vi "Test Gradient Control.vi"() -> ()   [LabVIEW 2015]
panel:
  in  "Frame Color":u32(colorbox)=16777216
  in  "Direction":T1(ring)
  in  "Slide":dbl(slide) scale=0.0..1.0
  in  "stop":bool
  in  "Color 2":u32(colorbox)
  in  "Color 1":u32(colorbox)
  out "Color Ramp":i32[][](graph)
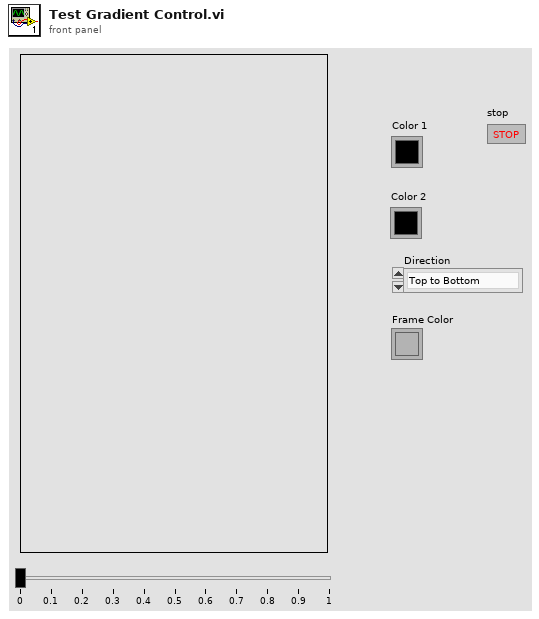
[diagram p1: front panel]
types:
  T1 = enum16{"Top to Bottom", "Bottom to Top", "Left to Right", "Right to Left"}
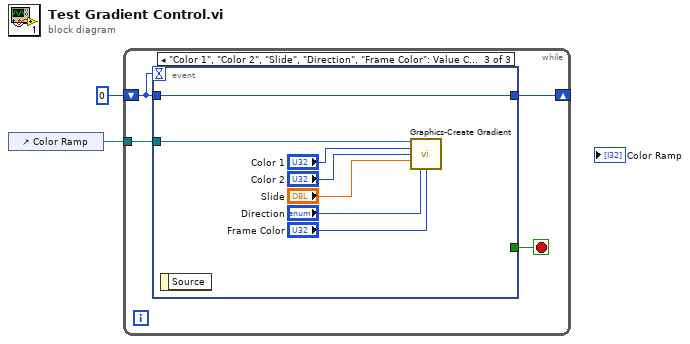
[diagram p0: block diagram]
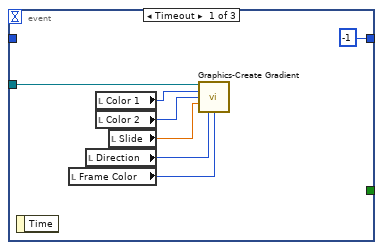
[diagram p2: hidden frame]
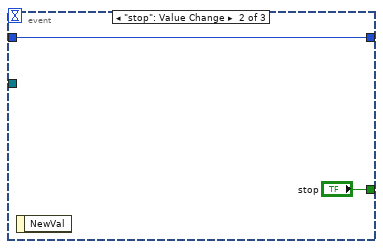
[diagram p3: hidden frame]
diagram:
  n1 = control-ref of="Color Ramp"() -> (w1:refnum<vi>)
  n2 = while {
    shift-right: [w4] -> _
    shift-left: 0 -> [w5]
    tunnel: w1 -> [w3]
    stop <- w6 stop-if-true
    n3 = event shown="[2] \"Color 1\", \"Color 2\", \"Slide\", \"Direction\", \"Frame Color\": Value Change" {
      selector: _ -> [_ _ _]
      dyn-events: _ -> [_ _ _]
      timeout: w5 -> [_ _ _]
      tunnel: [_ "stop" _] -> w6
      tunnel: w5 -> [_ w14 w22]
      tunnel: [-1 w14 w22] -> w4
      tunnel: w3 -> [w12 _ w21]
      event Timeout {
        n4 = event-data() -> ()  [unwired: 1 in, 1 out]
        n5 = local read "Frame Color"() -> (w7:u32)
        n6 = local read "Direction"() -> (w8:T1)
        n7 = local read "Color 1"() -> (w11:u32)
        n8 = local read "Color 2"() -> (w10:u32)
        n9 = local read "Slide"() -> (w9:dbl)
        n10 = call "Graphics-Create Gradient.vi"("intensity graph"=w12, "Color 1"=w11, "Color 2"=w10, "Fraction"=w9, "Direction"=w8, "Frame Color"=w7) -> ()  [unwired: 9 in, 1 out]
      }
      event "stop": Value Change {
        n11 = event-data() -> ()  [unwired: 1 in, 1 out]
      }
      event "Color 1", "Color 2", "Slide", "Direction", "Frame Color": Value Change {
        n12 = event-data() -> ()  [unwired: 1 in, 1 out]
        n13 = call "Graphics-Create Gradient.vi"("intensity graph"=w21, "Color 1"="Color 1", "Color 2"="Color 2", "Fraction"="Slide", "Direction"="Direction", "Frame Color"="Frame Color") -> ()  [unwired: 9 in, 1 out]
      }
    }
  }
